vi "Initialize.vi"(8 "error in (no error)":errorcluster, 11 "Stage_MadCityLabMicro in":refnum<class "Stage_MadCityLabMicro.lvclass">) -> (0 "error out":errorcluster, 3 "Stage_MadCityLabMicro out":refnum<class "Stage_MadCityLabMicro.lvclass">)   [LabVIEW 2020, in "Stage_MadCityLabMicro.lvlib" / "Stage_MadCityLabMicro.lvclass"]
uses:
  Stage_MadCityLabMicro.lvclass
  Dependency/MicroDrive.dll
  <vilib>/ActorFramework/Actor/Actor.lvclass
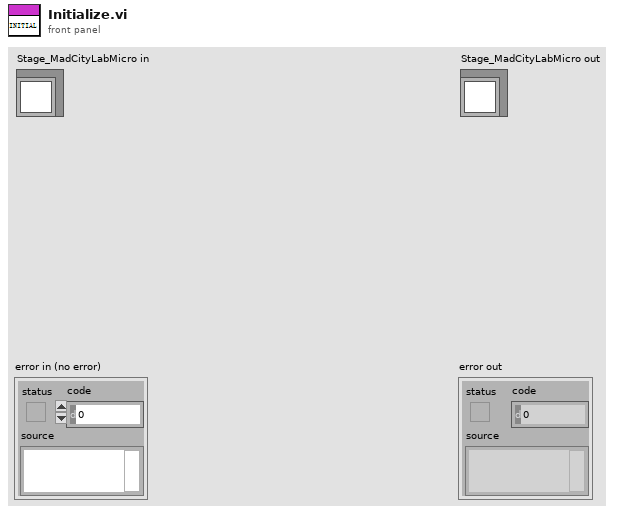
[diagram p1: front panel]
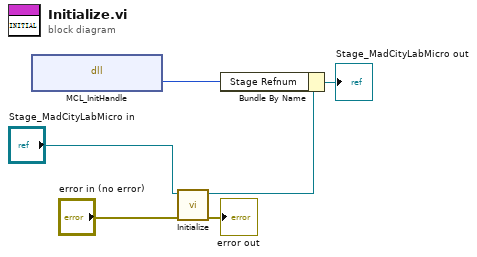
[diagram p0: block diagram]
diagram:
  n1 = dll-call lib="E:/Development/DevHardSoftware/MicroscopyFramework/Model/Hardware Layer/Real Hardware/Stage_MadCityLabMicro/Stage_MadCityLabMicro/Dependency/MicroDrive.dll" fn="MCL_InitHandle"() -> ("return type"=w4:i32)  [unwired: 3 in, 2 out]
  n2 = call-parent "Initialize.vi"("error in (no error)"="error in (no error)", "Device in"="Stage_MadCityLabMicro in") -> ("error out"=→"error out":errorcluster, "Device out"=w2:refnum<class "Stage_MadCityLabMicro.lvclass">)  [unwired: 8 in]
  n3 = Bundle By Name(cluster=w2, "Stage Refnum"=w4) -> (→"Stage_MadCityLabMicro out":refnum<class "Stage_MadCityLabMicro.lvclass">)
